vi "Existe_fichero_bandejas.vi"(8 "Error In":errorcluster) -> (0 "Error Out":errorcluster, 3 "existe fichero bandejas?":bool)   [LabVIEW 2019, in "SHARED VI'S.lvlib"]
uses:
  SHARED VI'S.lvlib
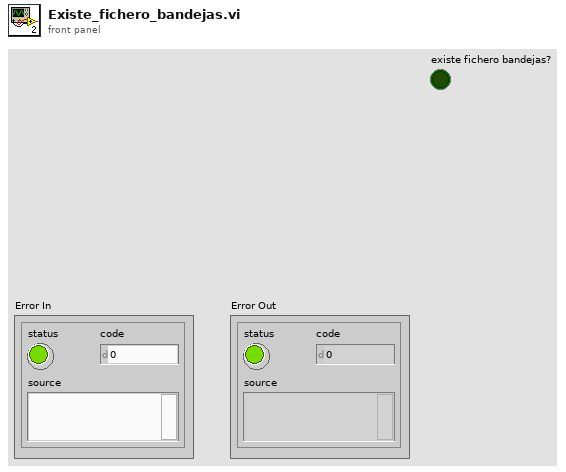
[diagram p1: front panel]
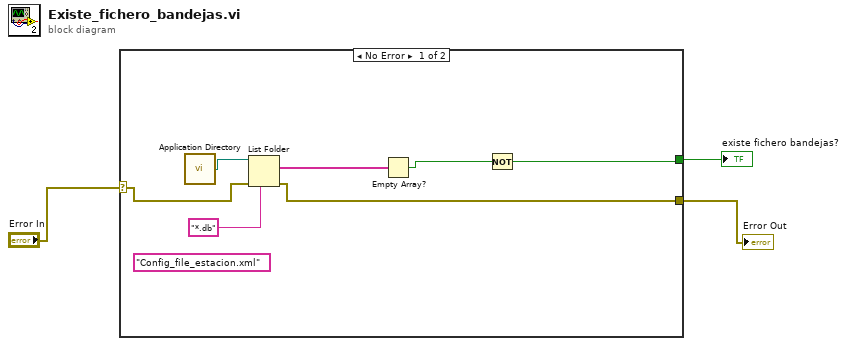
[diagram p0: block diagram]
diagram:
  n1 = case shown="No Error" "Error In" {
    selector: "Error In" -> [w9 w11]
    tunnel: [w6 w11] -> w2
    tunnel: [w4 _] -> w1
    frame No Error {
      (unwired) "Config_file_estacion.xml" ("name or relative path")
      n2 = call <vilib>:"Application Directory.vi"() -> ("Application Directory"=w10:path)
      n3 = List Folder(path=w10, pattern="*.db", error in=w9) -> (filenames=w7:string[], error out=w6:errorcluster)  [unwired: 1 in, 2 out]
      n4 = Empty Array?(array=w7) -> (empty?=w5:bool)
      n5 = Not(x=w5) -> (.not. x?=w4:bool)
    }
    frame Error {
    }
  }
  "Error Out" <- w2
  "existe fichero bandejas?" <- w1
